vi "Pose3d_TransformBy.vi"(9 "other Transform3d":T5={"TRANSLATION3D"={"X"=0.0, "Y"=0.0, "Z"=0.0}, "ROTATION3D"={"Q_quaternion"={"R"=1.0, "V"=[0.0, 0.0, 0.0]}}, "XF"=FALSE} {"TRANSLATION3D"."Z" format="%14.3f"; "TRANSLATION3D"."Y" format="%14.3f"; "TRANSLATION3D"."X" format="%14.3f"}, 11 "in Pose3d":T1={"Translation3d"={"X"=0.0, "Y"=0.0, "Z"=0.0}, "Rotation3d"={"Q_quaternion"={"R"=1.0, "V"=[0.0, 0.0, 0.0]}}} {"Translation3d"."Z" format="%14.3f"; "Translation3d"."Y" format="%14.3f"; "Translation3d"."X" format="%14.3f"}) -> (3 "out POSE3d":T1={"Translation3d"={"X"=0.0, "Y"=0.0, "Z"=0.0}, "Rotation3d"={"Q_quaternion"={"R"=1.0, "V"=[0.0, 0.0, 0.0]}}} {"Translation3d"."Z" format="%14.3f"; "Translation3d"."Y" format="%14.3f"; "Translation3d"."X" format="%14.3f"})   [LabVIEW 2019, in "Trajectory_Library.lvlib"]
doc: "Transforms the pose by the given transformation and returns the new transformed pose. \"plus\" is the same as \"transformBy\"\n\nParameters:\n - IN POSE3D - The input POSE data structure\n - OTHER TRANSFORM3D - The transform to transform the pose by.\n\nReturn:\n - OUT POSE3D - The transformed pose."
uses:
  Trajectory_Library.lvlib
  TypeDef/POSE3D.ctl
  TypeDef/TRANSLATION3D.ctl
  TypeDef/ROTATION3D.ctl
  TypeDef/QUATERNION.ctl
  TypeDef/TRANSFORM3D.ctl
  Translation3d_Create.vi
  Rotation3d_GetQuaterion.vi
  Quaternion_New.vi
  Quaternion_Times.vi
  Quaternion_Inverse.vi
  Quaternion_Get_All.vi
  Rotation3d_RotateBy.vi
  Rotation3d_Create_Quaternion.vi
  Quaternion_Normalize.vi
  Quaternion_New_Default.vi
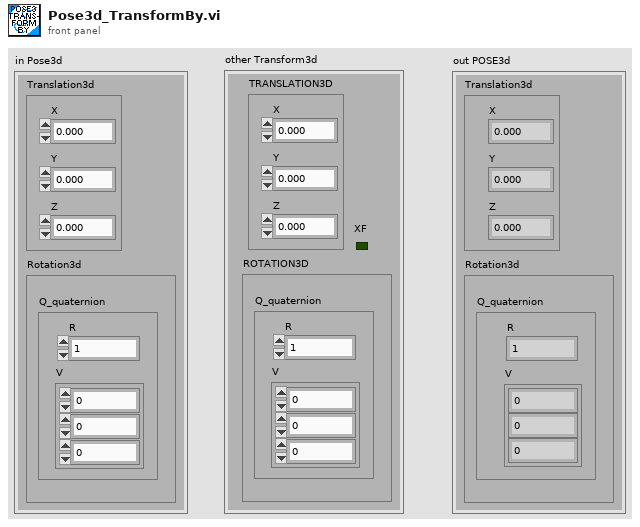
[diagram p1: front panel]
types:
  T1 = typedef "Trajectory_Library.lvlib/POSE3D.ctl" = cluster{"Translation3d":T2, "Rotation3d":T3}
  T2 = typedef "Trajectory_Library.lvlib/TRANSLATION3D.ctl" = cluster{"X":dbl, "Y":dbl, "Z":dbl}
  T3 = typedef "Trajectory_Library.lvlib/ROTATION3D.ctl" = cluster{"Q_quaternion":T4}
  T4 = typedef "Trajectory_Library.lvlib/QUATERNION.ctl" = cluster{"R":dbl, "V":dbl[]}
  T5 = typedef "Trajectory_Library.lvlib/TRANSFORM3D.ctl" = cluster{"TRANSLATION3D":T2, "ROTATION3D":T3, "XF":bool}
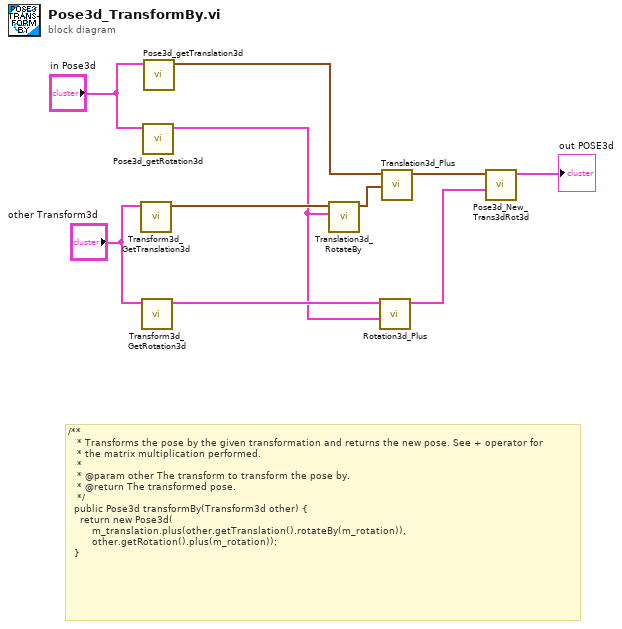
[diagram p0: block diagram]
diagram:
  # "/**\n   * Transforms the pose by the given transformation and returns the new pose. See + operator for\n   * the matrix multiplication performed.\n   *\n   * @param other The transform to transform the pose by.\n   * @return The transformed pose.\n   */\n  public Pose3d transformBy(Transform3d other) {\n    return new Pose3d(\n        m_translation.plus(other.getTranslation().rotateBy(m_rotation)),\n        other.getRotation().plus(m_rotation));\n  }"
  n1 = call "Transform3d_GetTranslation3d.vi"("in Transform3d"="other Transform3d") -> ("Translation3d"=w3:T2)  [unwired: 10 in]
  n2 = call "Transform3d_GetRotation3d.vi"("in Transform3d"="other Transform3d") -> ("Rotation3d"=w2:T3)  [unwired: 10 in]
  n3 = call "Pose3d_getRotation3d.vi"("in Pose3d"="in Pose3d") -> ("out Rotation3d"=w1:T3)  [unwired: 10 in]
  n4 = call "Pose3d_getTranslation3d.vi"("in Pose3d"="in Pose3d") -> ("out Translation3d"=w7:T2)  [unwired: 10 in]
  n5 = call "Translation3d_RotateBy.vi"("other Rot3d"=w1, "in Translation3D"=w3) -> ("out Translation3d"=w10:T2)  [unwired: 9 in]
  n6 = call "Rotation3d_Plus.vi"("other Rotation3d"=w1, "in Rotation3d"=w2) -> ("out Rotation3d"=w5:T3)  [unwired: 9 in]
  n7 = call "Translation3d_Plus.vi"("other Translation3d"=w10, "In Translation3d"=w7) -> ("Out Translation3d"=w6:T2)  [unwired: 9 in]
  n8 = call "Pose3d_New_Trans3dRot3d.vi"("Rotation3d"=w5, "Translation3d"=w6) -> ("outPose3d"=→"out POSE3d":T1)  [unwired: 9 in]
